vi "Frequence Domain Anlysis.vi"(8 "error in (no error)":errorcluster caption="错误输入（无错误）", 11 "采集信号输入":waveform(dbl)[](array[waveform])) -> (0 "error out":errorcluster caption="错误输出", 1 "THD Power Spectrum":cluster{"f0":dbl, "df":dbl, "magnitude":dbl[]}[](array[cluster]), 2 "detected fundamental frequency":dbl, 3 "S-Waveform Out":waveform(dbl), 4 "power spectrum":cluster{"f0":dbl, "df":dbl, "magnitude":dbl[]}, 5 "O-Waveform":waveform(dbl), 6 "Harmonics Data Out":dbl[](array[numeric]))   [LabVIEW 2019]
uses:
  <vilib>/measure/matone.llb/Harmonic Distortion Analyzer 1 Chan.vi
  <vilib>/measure/maspectr.llb/FFT Power Spectrum for 1 Chan.vi
  <vilib>/measure/maspectr.llb/FFT Power Spectrum for N Chan.vi
  <vilib>/measure/NI_MAPro.lvlib
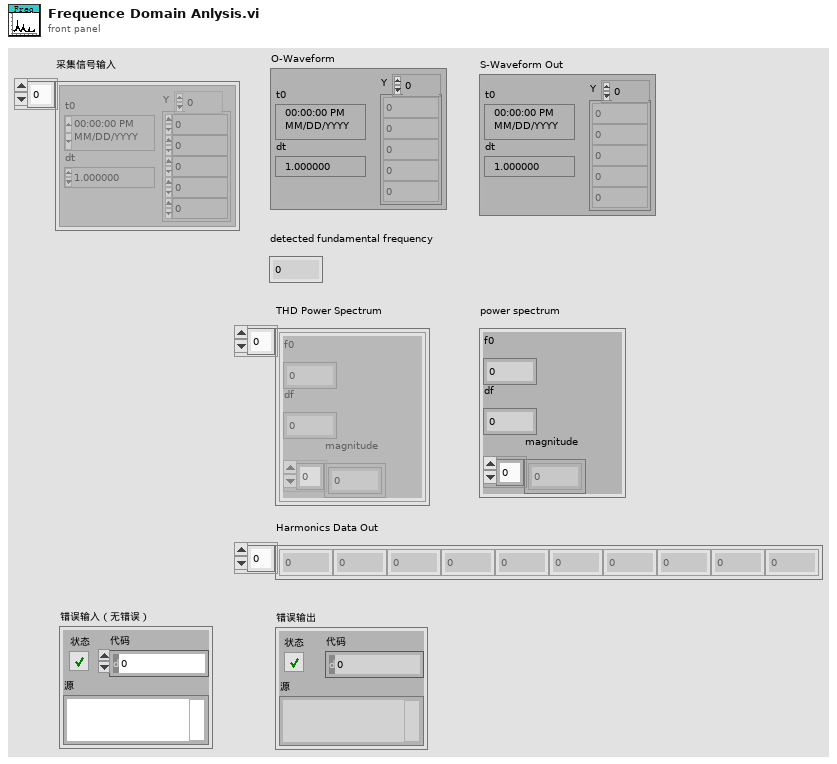
[diagram p1: front panel]
types:
  T1 = enum16{"None ", "Hanning", "Hamming", "Blackman-Harris", "Exact Blackman", "Blackman", "Flat Top", "4 Term B-Harris ", "7 Term B-Harris", "Low Sidelobe"}
  T2 = enum16{"none", "input signal", "fundamental signal", "residual signal", "harmonics only"}
  T3 = cluster{"approx freq. (optional)":dbl, "search (+/- % of Fsampl.)":dbl}
  T4 = cluster{"exported time signal":waveform(dbl), "exported spectrum (dB)":cluster{"f0":dbl, "df":dbl, "dB Spectrum (Hann)":dbl[]}}
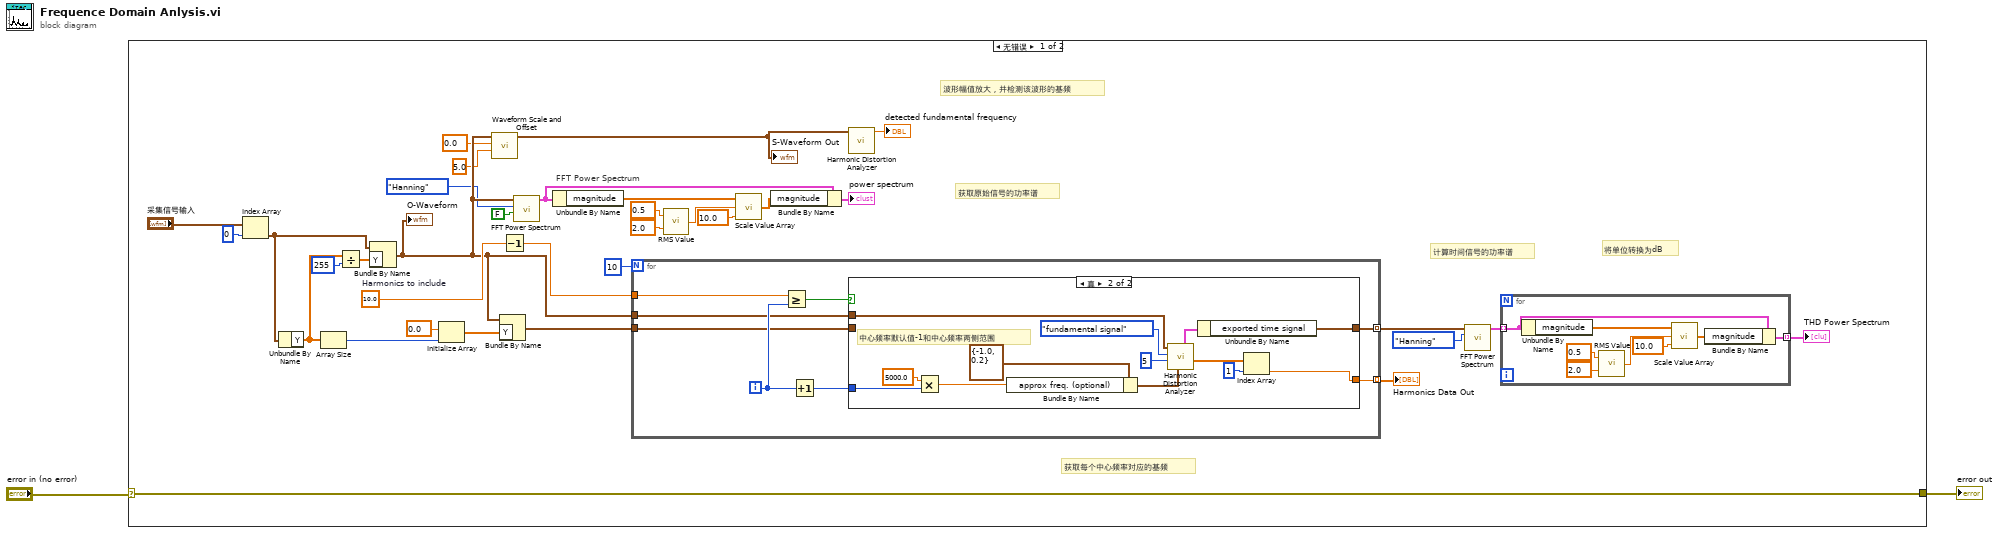
[diagram p0: block diagram]
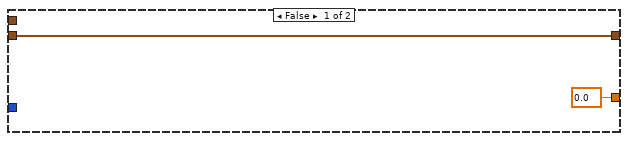
[diagram p2: hidden frame]
diagram:
  n1 = case shown="无错误" "error in (no error)" {
    selector: "error in (no error)" -> [w3 w68]
    tunnel: [w3 w68] -> w1
    frame No Error {
      w36 = 10.0  # Harmonics to include
      # "波形幅值放大，并检测该波形的基频"
      # "获取原始信号的功率谱"
      # "将单位转换为dB"
      # "计算时间信号的功率谱"
      # "获取每个中心频率对应的基频"
      # "FFT Power Spectrum"
      n2 = Index Array(array="采集信号输入", index=0) -> (element=w27:waveform(dbl))
      n3 = Unbundle By Name(w27) -> ("Y"=w18:dbl[])
      n4 = Array Size(array=w18) -> (size(s)=w6:i32)
      n5 = Divide(x=w18, y=255) -> (x/y=w8:dbl[])
      n6 = Bundle By Name(cluster=w27, "Y"=w8) -> (w30:waveform(dbl))
      "O-Waveform" <- w30
      n7 = Initialize Array(0.0 ("element"), w6) -> (w19:dbl[])
      n8 = call <vilib>:"Waveform Scale and Offset.vi"("scale"=5.0, "offset"=0.0, "waveform in"=w30) -> ("waveform out"=w32:waveform(dbl))  [unwired: 7 in, 1 out]
      "S-Waveform Out" <- w32
      n9 = Bundle By Name(cluster=w30, "Y"=w19) -> (w20:waveform(dbl))
      n10 = Decrement(x=w36) -> (x-1=w22:dbl)
      n11 = call-poly <vilib>:"FFT Power Spectrum.vi"("dB On (F)"=FALSE, "window"=T1."Hanning", "time signal"=w30) -> ("power spectrum"=w13:cluster{"f0":dbl, "df":dbl, "magnitude":dbl[]})  [unwired: 5 in, 3 out]
      n12 = Unbundle By Name(w13) -> ("magnitude"=w23:dbl[])
      n13 = for {
        N: 10 -> [_]
        tunnel: [w49] -> w12 mode=indexing
        tunnel: w30 -> [w48]
        tunnel: [w50] -> w31 mode=indexing
        tunnel: w20 -> [w47]
        tunnel: w22 -> [w45]
        i -> [w51]
        n14 = Greater Or Equal?(x=w45, y=w51) -> (x >= y?=w46:bool)
        n15 = Increment(x=w51) -> (x+1=w52:i32)
        n16 = case shown="真" w46 {
          tunnel: w52 -> [_ w65]
          tunnel: [0.0 ("Numeric") w64] -> w50
          tunnel: [w54 w55] -> w49
          tunnel: w48 -> [_ w58]
          tunnel: w47 -> [w54 _]
          frame False {
          }
          frame True {
            # "中心频率默认值-1和中心频率两侧范围"
            n17 = Multiply(x=5000.0 ("frequency (Hz)"), y=w65) -> (x*y=w61:dbl)
            n18 = Bundle By Name(cluster=T3 {"approx freq. (optional)"=-1.0, "search (+/- % of Fsampl.)"=0.2} ("advanced search"), "approx freq. (optional)"=w61) -> (w66:T3)
            n19 = call-poly <vilib>:"Harmonic Distortion Analyzer.vi"("advanced search"=w66, "highest harmonic"=5, "export mode"=T2."fundamental signal" ("export signals"), "signal in"=w58) -> ("components level"=w63:dbl[], "exported signals"=w56:T4)  [unwired: 2 in, 4 out]
            n20 = Unbundle By Name(w56) -> ("exported time signal"=w55:waveform(dbl))
            n21 = Index Array(array=w63, index=1) -> (element=w64:dbl)
          }
        }
      }
      "Harmonics Data Out" <- w31
      n22 = call "RMS Value.vi"("y"=2.0, "y 2"=0.5 ("y")) -> ("Numeric"=w24:dbl)
      n23 = call "Scale Value Array.vi"("y"=10.0, "Numeric"=w24, "magnitude 2"=w23) -> ("magnitude"=w26:dbl[])
      n24 = Bundle By Name(cluster=w13, "magnitude"=w26) -> (→"power spectrum":cluster{"f0":dbl, "df":dbl, "magnitude":dbl[]})
      n25 = call-poly <vilib>:"Harmonic Distortion Analyzer.vi"("signal in"=w32) -> ("detected fundamental frequency"=→"detected fundamental frequency":dbl)  [unwired: 5 in, 5 out]
      n26 = call-poly <vilib>:"FFT Power Spectrum.vi"("window"=T1."Hanning", "time signals"=w12) -> ("power spectra"=w10:cluster{"f0":dbl, "df":dbl, "magnitude":dbl[]}[])  [unwired: 6 in, 3 out]
      n27 = for {
        tunnel: w10 -> [w42] mode=indexing
        tunnel: [w43] -> w34 mode=indexing
        n28 = Unbundle By Name(w42) -> ("magnitude"=w41:dbl[])
        n29 = call "RMS Value.vi"("y"=2.0, "y 2"=0.5 ("y")) -> ("Numeric"=w37:dbl)
        n30 = call "Scale Value Array.vi"("y"=10.0, "Numeric"=w37, "magnitude 2"=w41) -> ("magnitude"=w40:dbl[])
        n31 = Bundle By Name(cluster=w42, "magnitude"=w40) -> (w43:cluster{"f0":dbl, "df":dbl, "magnitude":dbl[]})
      }
      "THD Power Spectrum" <- w34
    }
    frame Error {
    }
  }
  "error out" <- w1
